vi "04齿轮轴批次号上传.vi"(2 "齿轮轴批次号":string) -> ()   [LabVIEW 2013]
uses:
  <vilib>/Utility/error.llb/whitespace.ctl
panel:
  in  "error in (no error)":errorcluster
  out "error out":errorcluster
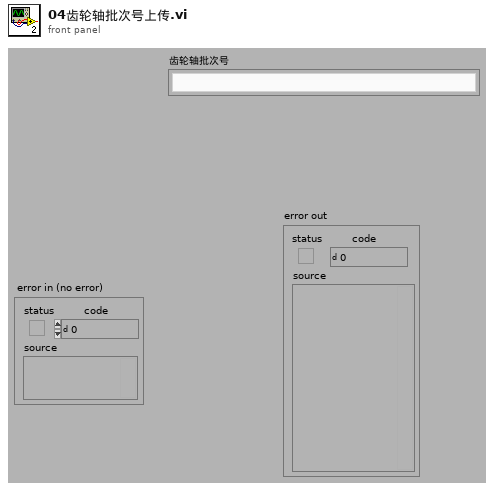
[diagram p1: front panel]
types:
  T1 = typedef "whitespace.ctl" = u16
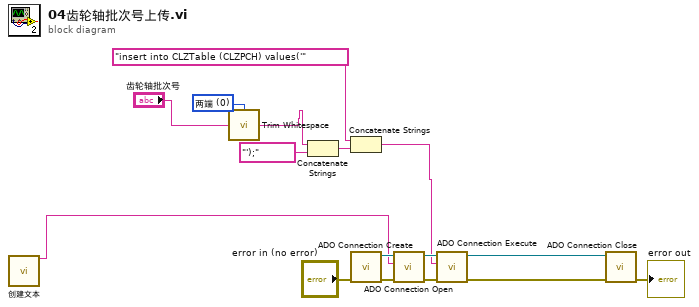
[diagram p0: block diagram]
diagram:
  w5 = T1 0 items=["两端", "字符串首端", "字符串末端"] ("location (both)")
  n1 = call "创建文本"() -> ("Result"=w2:string)  [unwired: 14 in, 1 out]
  n2 = call <vilib>:"Trim Whitespace.vi"("string"="齿轮轴批次号", "location (both)"=w5) -> ("trimmed string"=w3:string)
  n3 = Concatenate Strings(w3, "');" ("字符串")) -> (w6:string)
  n4 = Concatenate Strings("insert into CLZTable (CLZPCH) values('" ("字符串"), w6) -> (w1:string)
  n5 = call "ADO Connection Create.vi"("error in (no error)"="error in (no error)") -> ("error out"=w15:errorcluster, "ADODB._Connection Out"=w16:refnum<k7>)  [unwired: 9 out]
  n6 = call "ADO Connection Open.vi"("error in (no error)"=w15, "ConnectionString"=w2, "ADODB._Connection In"=w16) -> ("error out"=w14:errorcluster, "ADODB._Connection Out"=w13:refnum<k7>)  [unwired: 7 out]
  n7 = call "ADO Connection Execute.vi"("error in (no error)"=w14, "CommandText"=w1, "ADODB._Connection In"=w13) -> ("error out"=w8:errorcluster, "ADODB._Connection Out"=w12:refnum<k7>)  [unwired: 7 out]
  n8 = call "ADO Connection Close.vi"("error in (no error)"=w8, "ADODB._Connection In"=w12) -> ("error out"=→"error out":errorcluster)  [unwired: 9 out]
